vi "Read Data.vi"(8 "error in":errorcluster, 11 "Serial in":refnum<class "Serial.lvclass">) -> (0 "error out":errorcluster, 2 "Data Read":string, 3 "Serial out":refnum<class "Serial.lvclass">)   [LabVIEW 2021, in "Serial.lvclass"]
uses:
  Serial.lvclass
  Serial.lvclass/Serial.ctl
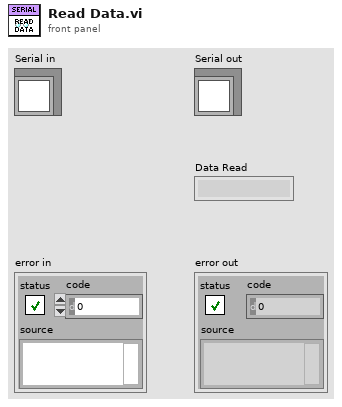
[diagram p1: front panel]
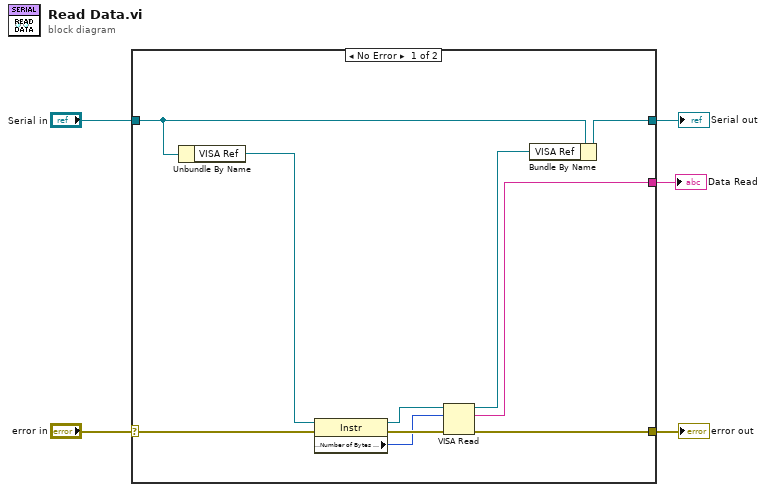
[diagram p0: block diagram]
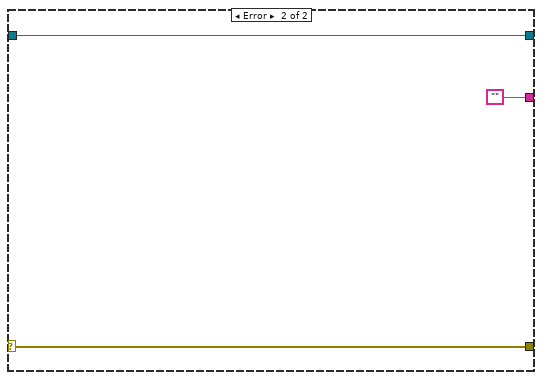
[diagram p2: hidden frame]
diagram:
  n1 = case shown="No Error" "error in" {
    selector: "error in" -> [w12 w17]
    tunnel: "Serial in" -> [w14 w16]
    tunnel: [w7 w16] -> w4
    tunnel: [w15 w17] -> w2
    tunnel: [w8 ""] -> w1
    frame No Error {
      n2 = Unbundle By Name(w14) -> ("VISA Ref"=w13:refnum<visa-resource-name>)
      n3 = property class="Instr"(reference=w13, error in=w12) -> (reference out=w9:refnum<visa-resource-name>, error out=w11:errorcluster, "Serial Settings:Number of Bytes at Serial Port"=w10:u32)
      n4 = VISA Read(VISA resource name=w9, byte count=w10, error in (no error)=w11) -> (VISA resource name out=w6:refnum<visa-resource-name>, read buffer=w8:string, error out=w15:errorcluster)  [unwired: 1 out]
      n5 = Bundle By Name(cluster=w14, "VISA Ref"=w6) -> (w7:refnum<class "Serial.lvclass">)
    }
    frame Error {
    }
  }
  "error out" <- w2
  "Serial out" <- w4
  "Data Read" <- w1
